vi "Get Terminals.vi"(8 "error in (no error)":errorcluster, 10 "to object reference":i32, 11 "Data Cluster in":T1) -> (0 "error out":errorcluster, 2 "Terms[]":refnum<vi>[](array[refnum]), 3 "Data Cluster out":T1)   [LabVIEW 2025, in "Scripting Server.lvlib"]
uses:
  Scripting Server.lvlib
  Module Data--cluster.ctl
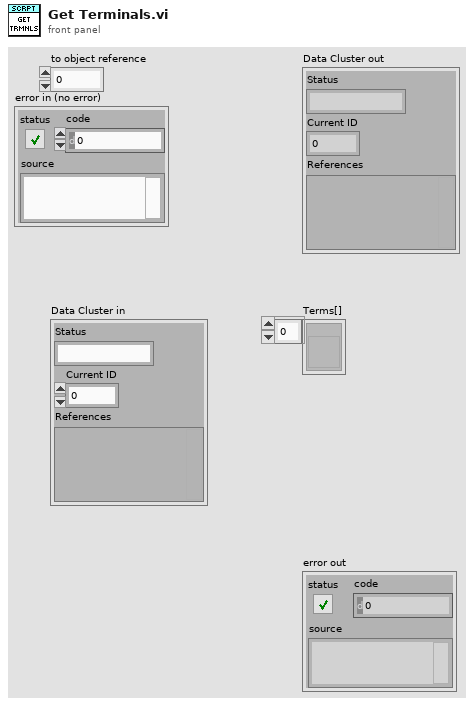
[diagram p1: front panel]
types:
  T1 = typedef "Scripting Server.lvlib/Module Data--cluster.ctl" = cluster{"Status":string, "Current ID":i32, "References":variant}
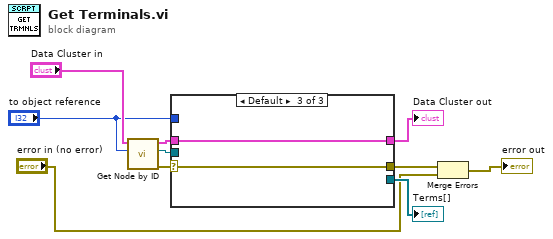
[diagram p0: block diagram]
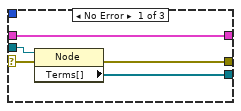
[diagram p2: hidden frame]
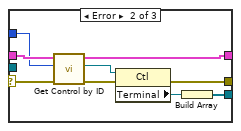
[diagram p3: hidden frame]
diagram:
  n1 = call "Get Node by ID.vi"("ID"="to object reference", "Data Cluster in"="Data Cluster in") -> ("error out"=w6:errorcluster, "specific class reference"=w9:refnum<vi>, "Data Cluster out"=w5:T1)  [unwired: 7 in]
  n2 = case shown="Default" w6 {
    selector: w6 -> [w12 w24 w26]
    tunnel: [w15 w19 w26] -> w10
    tunnel: w9 -> [w14 _ _]
    tunnel: [w13 w16 _] -> w7
    tunnel: w5 -> [w11 w22 w25]
    tunnel: [w11 w21 w25] -> w4
    tunnel: "to object reference" -> [_ w20 _]
    frame No Error {
      n3 = property class="Node"(reference=w14, error in=w12) -> (error out=w15:errorcluster, "Terms[]"=w13:refnum<vi>[])  [unwired: 1 out]
    }
    frame Error {
      n4 = call "Get Control by ID.vi"("error in (no error)"=w24, "ID"=w20, "Data Cluster in"=w22) -> ("error out"=w23:errorcluster, "specific class reference"=w18:refnum<vi>, "Data Cluster out"=w21:T1)  [unwired: 6 in]
      n5 = property class="Ctl"(reference=w18, error in=w23) -> (error out=w19:errorcluster, "Terminal"=w17:refnum<vi>)  [unwired: 1 out]
      n6 = Build Array(w17) -> (w16:refnum<vi>[])
    }
    frame Default {
    }
  }
  "Data Cluster out" <- w4
  "Terms[]" <- w7
  n7 = Merge Errors(w10, "error in (no error)") -> (→"error out":errorcluster)
